vi "Create Configuration Data.vi"(8 "error in (no error)":errorcluster, 11 "Item Ref in":T1 format="%.0x") -> (0 "error out":errorcluster, 3 "Item Ref out":T1 format="%.0x")   [LabVIEW 2017, in "DSF System Explorer.lvlib"]
uses:
  DSF System Explorer.lvlib
  <vilib>/NI Veristand/Custom Device API/Custom Device Item Ref.ctl
  DSF Core.lvlibp/Typedefs/DSF Engine Framework Configuration.ctl
  DSF Core.lvlibp/Typedefs/DSF Engine Plugin Configuration.ctl
  DSF Core.lvlibp/Typedefs/DSF Core Plugin Configuration.ctl
  DSF Core.lvlibp/Typedefs/DSF Timing Info.ctl
  DSF Core.lvlibp/Typedefs/DSF Settings Info.ctl
  DSF Core.lvlibp/Typedefs/DSF Version Info.ctl
  DSF Core.lvlibp/Typedefs/DSF Engine Plugin Thread Configuration.ctl
  DSF Core.lvlibp/Typedefs/DSF Core Thread Configuration.ctl
  DSF Core.lvlibp/Typedefs/DSF Engine Transfer Group Configuration.ctl
  DSF Core.lvlibp/Typedefs/DSF Core Group Configuration.ctl
  DSF Core.lvlibp/Typedefs/DSF Direction.ctl
  DSF Core.lvlibp/Typedefs/DSF Timeout Behavior.ctl
  DSF Core.lvlibp/Typedefs/DSF Engine Transfer Configuration.ctl
  DSF Core.lvlibp/Typedefs/DSF Core Transfer Configuration.ctl
  DSF Core.lvlibp/Typedefs/DSF Engine Channel Configuration.ctl
  DSF Core.lvlibp/Typedefs/DSF Core Channel Configuration.ctl
  DSF Core.lvlibp/Typedefs/DSF Data Type.ctl
  <vilib>/NI Veristand/Custom Device API/Set Item Property (U32).vi
  DSF Core.lvlibp
  <vilib>/NI Veristand/Custom Device API/Custom Device API.lvlib
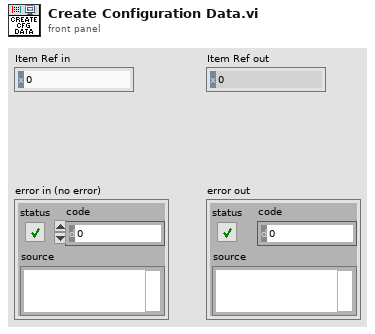
[diagram p1: front panel]
types:
  T1 = typedef "Custom Device API.lvlib/Custom Device Item Ref.ctl" = u64
  T2 = typedef "DSF Core.lvlibp/DSF Engine Framework Configuration.ctl" = cluster{"plugins":T3[]}
  T3 = typedef "DSF Core.lvlibp/DSF Engine Plugin Configuration.ctl" = cluster{"core":T4, "component settings":T6[], "threads":T8[]}
  T4 = typedef "DSF Core.lvlibp/DSF Core Plugin Configuration.ctl" = cluster{"name":string, "components":string[], "cycle timing":T5}
  T5 = typedef "DSF Core.lvlibp/DSF Timing Info.ctl" = cluster{"priority":u64, "decimation":u64, "offset":u64}
  T6 = typedef "DSF Core.lvlibp/DSF Settings Info.ctl" = cluster{"component":string, "version":T7, "values":cluster{"key":string, "value":string}[]}
  T7 = typedef "DSF Core.lvlibp/DSF Version Info.ctl" = cluster{"major":u32, "minor":u32, "fix":u32, "build":string}
  T8 = typedef "DSF Core.lvlibp/DSF Engine Plugin Thread Configuration.ctl" = cluster{"core":T9, "component settings":T6[], "transfer groups":T10[]}
  T9 = typedef "DSF Core.lvlibp/DSF Core Thread Configuration.ctl" = cluster{"processor":i32, "priority offset":i16}
  T10 = typedef "DSF Core.lvlibp/DSF Engine Transfer Group Configuration.ctl" = cluster{"core":T11, "component settings":T6[], "transfers":T14[]}
  T11 = typedef "DSF Core.lvlibp/DSF Core Group Configuration.ctl" = cluster{"name":string, "direction":T12, "cycle timing":T5, "timeout behavior":T13}
  T12 = typedef "DSF Core.lvlibp/DSF Direction.ctl" = enum8{"Tx", "Rx"}
  T13 = typedef "DSF Core.lvlibp/DSF Timeout Behavior.ctl" = enum8{"Increment Late Count", "Throw Error"}
  T14 = typedef "DSF Core.lvlibp/DSF Engine Transfer Configuration.ctl" = cluster{"core":T15, "component settings":T6[], "channels":T16[]}
  T15 = typedef "DSF Core.lvlibp/DSF Core Transfer Configuration.ctl" = cluster{"name":string}
  T16 = typedef "DSF Core.lvlibp/DSF Engine Channel Configuration.ctl" = cluster{"core":T17, "component settings":T6[]}
  T17 = typedef "DSF Core.lvlibp/DSF Core Channel Configuration.ctl" = cluster{"name":string, "units":string, "engine data type":T18, "string data type":T18, "string offset":u64}
  T18 = typedef "DSF Core.lvlibp/DSF Data Type.ctl" = enum8{"Bool", "SGL", "DBL", "I8", "I16", "I32", "I64", "U8", "U16", "U32", "U64"}
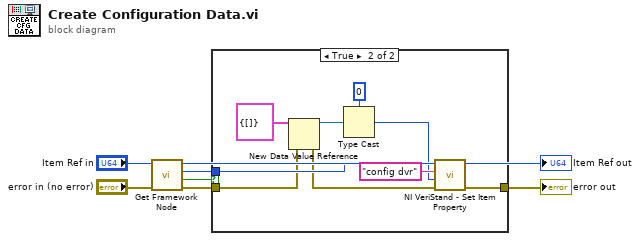
[diagram p0: block diagram]
diagram:
  n1 = call "Get Framework Node.vi"("error in (no error)"="error in (no error)", "Item Ref in"="Item Ref in") -> ("error out"=w5:errorcluster, "found?"=w2:bool, "Framework Ref"=w4:T1, "Item Ref out"=→"Item Ref out":T1)  [unwired: 6 in]
  n2 = case shown="True" w2 {
    tunnel: w5 -> [w8 w11]
    tunnel: w4 -> [_ w16]
    tunnel: [w8 w15] -> w3
    frame False {
    }
    frame True {
      n3 = New Data Value Reference(data value=T2 {"plugins"=[]} ("framework configuration"), error in=w11) -> (data value reference=w13:refnum<data-value>, error out=w10:errorcluster)
      n4 = Type Cast(type=u32 0, x=w13) -> (*(type *) &x=w9:u32)
      n5 = call-poly <vilib>:"NI VeriStand - Set Item Property.vi"("error in (no error)"=w10, "Value"=w9, "Property Name"="config dvr", "Item Ref in"=w16) -> ("error out"=w15:errorcluster)  [unwired: 5 in, 2 out]
    }
  }
  "error out" <- w3
